vi "Test Loopback.vi"() -> ()   [LabVIEW 2011]
panel:
  out "decimal integer string":string
  in  "stop":bool
  in  "Machine":string="localhost"
  in  "Port":u16=6341
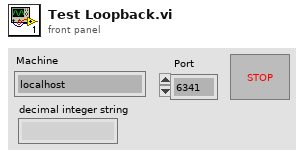
[diagram p1: front panel]
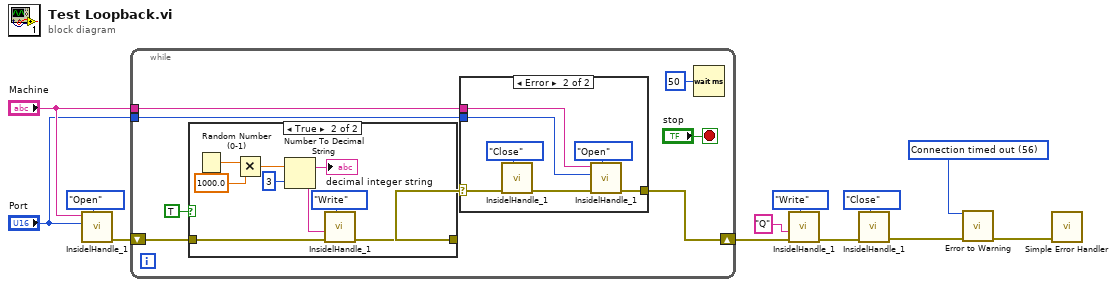
[diagram p0: block diagram]
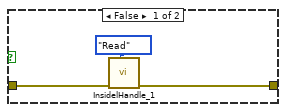
[diagram p2: hidden frame]
diagram:
  w3 = 56 items=["No Error", "Argument Error", "Memory Full", "Out of Zone", "End of File", "File Already Open", "Generic File IO Error", "File Not Found", "File Permission Error", "Disk Full", "Duplicate Path", "Too Many Files Open", "Not Enabled", "Resource File Not Found", "Cannot Add Resource", "Resource Not Found", "Image Not Found", "Image Memory Error", "Pen Does Not Exist", "Config Bad Type", "Config Token Not Found", "Config Parse Error", "Config Memory Error", "Bad External Code Format", "Bad External Code Offset", "External Code Not Present", "Null Window", "Destroy Window Mixup", "Null Menu", "Print Aborted", "Bad Print Record", "Print Driver Error", "Windows Error During Print", "Memory Error During Print", "Print Dialog Error", "Generic Print Error", "Invalid Device Refnum", "Device Not Found", "Device Parameter Error", "Device Unit Error", "Can't Open Device", "Device Call Aborted", "Generic Error", "Cancelled By User", "Object ID Too Low", "Object ID Too High", "Object Not In Heap", "Unknown Heap", "Bad DefProc ID", "DefProc Not In Table", "Message Out Of Range", "Null Method", "Unknown Message", "Manager Call Not Supported", "Bad address", "Connection In progress", "Connection timed out", "Connection is already in progress", "Network attribute not supported", "Network error", "Address in use", "System out of memory", "Connection aborted", "Connection refused", "Connection is not connected", "Connection is already connected", "Connection closed", "Initialize error (interapplication manager)", "Bad occurrence", "Wait on unbound occurrence handler", "Occurrence queue overflow", "Bad path", "Semaphore not signaled", "Unrecognized type (interapplication manager)"] ("1st Error to Convert")
  n1 = call "InsidelHandle_1.vi"("Mode"=enum16{"Open", "Read", "Write", "Close"}."Open", "Port"="Port", "Machine"="Machine") -> ("error out"=w11:errorcluster)  [unwired: 7 in, 1 out]
  n2 = while {
    shift-right: [w19] -> w7
    shift-left: w11 -> [w18]
    tunnel: "Machine" -> [w16]
    tunnel: "Port" -> [w15]
    stop <- "stop" stop-if-true
    n3 = case shown="True" TRUE {
      tunnel: w18 -> [w22 w31]
      tunnel: [w21 w30] -> w17
      frame False {
        n4 = call "InsidelHandle_1.vi"("Mode"=enum16{"Open", "Read", "Write", "Close"}."Read", "error in (no error)"=w22) -> ("error out"=w21:errorcluster)  [unwired: 8 in, 1 out]
      }
      frame True {
        n5 = Random Number (0-1)() -> (number: 0 to 1=w26:dbl)
        n6 = Multiply(x=w26, y=1000.0) -> (x*y=w24:dbl)
        n7 = Number To Decimal String(number=w24, width (-)=i16 3) -> (decimal integer string=w27:string)
        "decimal integer string" <- w27
        n8 = call "InsidelHandle_1.vi"("Mode"=enum16{"Open", "Read", "Write", "Close"}."Write", "error in (no error)"=w31, "data in"=w27) -> ("error out"=w30:errorcluster)  [unwired: 7 in, 1 out]
      }
    }
    n9 = case shown="Error" w17 {
      selector: w17 -> [w32 w35]
      tunnel: [w32 w36] -> w19
      tunnel: w16 -> [_ w34]
      tunnel: w15 -> [_ w33]
      frame No Error {
      }
      frame Error {
        n10 = call "InsidelHandle_1.vi"("Mode"=enum16{"Open", "Read", "Write", "Close"}."Close", "error in (no error)"=w35) -> ("error out"=w37:errorcluster)  [unwired: 8 in, 1 out]
        n11 = call "InsidelHandle_1.vi"("Mode"=enum16{"Open", "Read", "Write", "Close"}."Open", "error in (no error)"=w37, "Port"=w33, "Machine"=w34) -> ("error out"=w36:errorcluster)  [unwired: 6 in, 1 out]
      }
    }
    n12 = Wait (ms)(milliseconds to wait=u32 50) -> ()  [unwired: 1 out]
  }
  n13 = call "InsidelHandle_1.vi"("Mode"=enum16{"Open", "Read", "Write", "Close"}."Write", "error in (no error)"=w7, "data in"="Q") -> ("error out"=w8:errorcluster)  [unwired: 7 in, 1 out]
  n14 = call "InsidelHandle_1.vi"("Mode"=enum16{"Open", "Read", "Write", "Close"}."Close", "error in (no error)"=w8) -> ("error out"=w2:errorcluster)  [unwired: 8 in, 1 out]
  n15 = call <vilib>:"Error to Warning.vi"("1st Error to Convert"=w3, "error in"=w2) -> ("warning out"=w1:errorcluster)  [unwired: 3 in, 10 out]
  n16 = call <vilib>:"Simple Error Handler.vi"("error in (no error)"=w1) -> ()  [unwired: 1 in, 8 out]
